vi "New Tree Handle.vi"(8 "error in (no error)":errorcluster, 11 "Delimiter (\\)":string="\\") -> (0 "error out":errorcluster, 3 "Tree Map Handle Out":T1)   [LabVIEW 2020, in "Blue Tree Map OpenSource.lvlib"]
doc: "Use this VI to initialize a new Tree Map Handle.\n\nYou must declare a delimiter when opening a new handle.\nThe delimiter will be used when exporting the tree map to a LabVIEW tree control. The LabVIEW tree control uses the delimiter to separate tree path names.\nTree path names will NOT be allowed to contain the specified delimiter. So, choose wisely."
uses:
  Blue Tree Map OpenSource.lvlib
  Typedefs/Tree Map Handle.ctl
  Typedefs/Tree Map.ctl
  Typedefs/Tree Map Data.ctl
  Typedefs/Tree Node Data.ctl
  Typedefs/Attribute Map.ctl
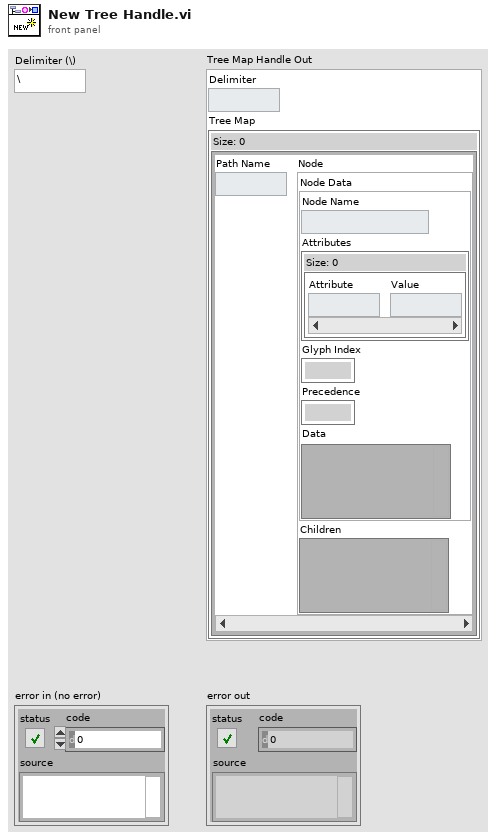
[diagram p1: front panel]
types:
  T1 = typedef "Blue Tree Map OpenSource.lvlib/Tree Map Handle.ctl" = cluster{"Delimiter":string, "Tree Map":T2}
  T2 = typedef "Blue Tree Map OpenSource.lvlib/Tree Map.ctl" = map{string, T3}
  T3 = typedef "Blue Tree Map OpenSource.lvlib/Tree Map Data.ctl" = cluster{"Node Data":T4, "Children":variant}
  T4 = typedef "Blue Tree Map OpenSource.lvlib/Tree Node Data.ctl" = cluster{"Node Name":string, "Attributes":T5, "Glyph Index":i32, "Precedence":i32, "Data":variant}
  T5 = typedef "Blue Tree Map OpenSource.lvlib/Attribute Map.ctl" = map{string, string}
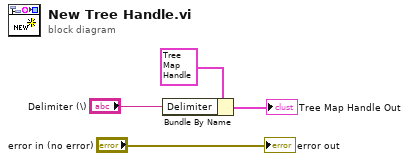
[diagram p0: block diagram]
diagram:
  n1 = Bundle By Name(cluster=T1 {"Delimiter"="", "Tree Map"={}} ("Tree Map Handle Out"), "Delimiter"="Delimiter (\\)") -> (→"Tree Map Handle Out":T1)
  "error out" <- "error in (no error)"
